vi "CSDB_SVEdit.load SV CSV file.vi"(1 "CSVPath":path, 5 "error in":errorcluster) -> (15 "SVValues":string[][](array[string]), 16 "SVHeader":string[](array[string]), 19 "error out":errorcluster)   [LabVIEW 2014, in "CSDB_SVEdit.lvlib"]
doc: "Loads the header and the values of a Shared Variable configuration from a CSV file."
uses:
  CSDB_SVEdit.lvlib
  CSlibraries/UtilityLib/UtilityLib.lvlib
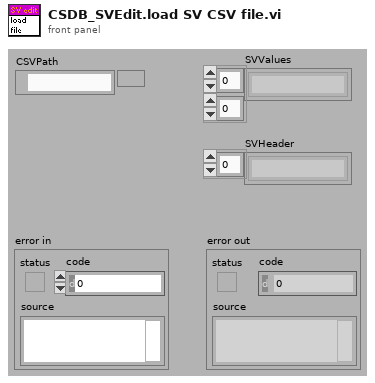
[diagram p1: front panel]
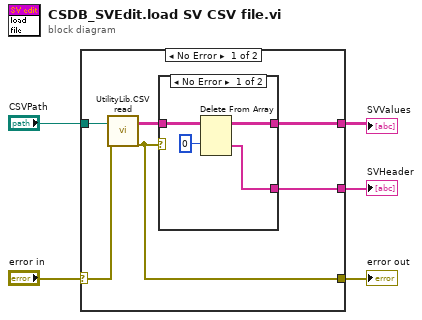
[diagram p0: block diagram]
diagram:
  n1 = case shown="No Error" "error in" {
    selector: "error in" -> [w6 w16]
    tunnel: [w11 _] -> w5
    tunnel: [w10 _] -> w4
    tunnel: [w9 w16] -> w3
    tunnel: "CSVPath" -> [w7 _]
    frame No Error {
      n2 = call "UtilityLib.CSV read.vi"("file (use dialog)"=w7, "error in"=w6) -> ("CSVArray"=w8:string[][], "error out"=w9:errorcluster)  [unwired: 16 in]
      n3 = case shown="No Error" w9 {
        tunnel: w8 -> [w14 _]
        tunnel: [w13 _] -> w10
        tunnel: [w12 _] -> w11
        frame No Error {
          n4 = Delete From Array(array=w14, index (row)=0) -> (deleted portion=w12:string[], array with subset deleted=w13:string[][])  [unwired: 2 in]
        }
        frame Error {
        }
      }
    }
    frame Error {
    }
  }
  "SVHeader" <- w5
  "SVValues" <- w4
  "error out" <- w3
